vi "Update Boolean.vi"(8 "error in (no error)":errorcluster, 10 "Boolean":bool, 11 "Indicators in":refnum<class "Indicators.lvclass">) -> (0 "error out":errorcluster, 3 "Indicators out":refnum<class "Indicators.lvclass">)   [LabVIEW 2020, in "Indicators.lvlib" / "Indicators.lvclass"]
uses:
  Indicators.lvclass
  Indicators.lvclass/Indicators.ctl
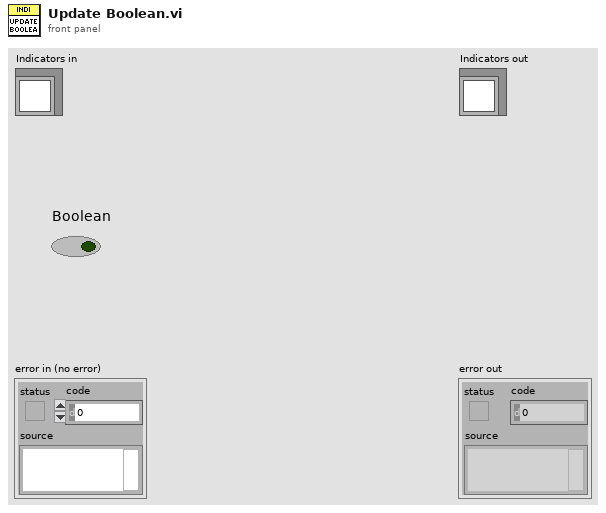
[diagram p1: front panel]
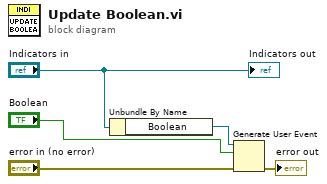
[diagram p0: block diagram]
diagram:
  n1 = Unbundle By Name("Indicators in") -> ("Boolean"=w2:refnum<user-event>)
  n2 = Generate User Event(user event=w2, event data cluster="Boolean", error in="error in (no error)") -> (error out=→"error out":errorcluster)  [unwired: 1 in, 1 out]
  "Indicators out" <- "Indicators in"
